vi "AddAutoMode.vi"(7 "error in (no error)":errorcluster, 9 "Autonomous Mode":string, 10 "Table Prefix":string="330AutonomousSelector") -> (0 "error out":errorcluster)   [LabVIEW 2012, in "AutonomousSelector.lvlib"]
doc: "Adds a single Autonomous Mode to the Autonomous Selector on the Dashboard. \n\n<B>Table Prefix</B> The Sub Table in Network Tables. The data will be stored in /SmartDashboard/<Table Prefix>\n<B>Autonomous Mode</B> The name of the Autonomous Mode to add"
uses:
  AutonomousSelector.lvlib
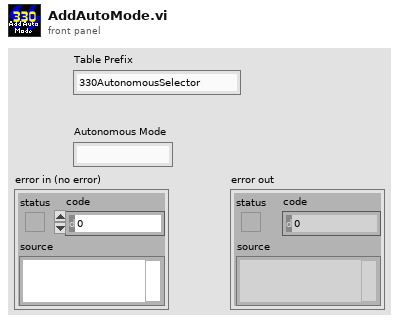
[diagram p1: front panel]
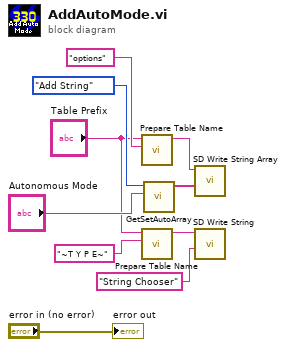
[diagram p0: block diagram]
diagram:
  n1 = call <vilib>:"Prepare Table Name.vi"("Name"="options", "Table Prefix"="Table Prefix") -> ("Prefixed Name"=w9:string)  [unwired: 9 in]
  n2 = call <vilib>:"Prepare Table Name.vi"("Name"="~T Y P E~", "Table Prefix"="Table Prefix") -> ("Prefixed Name"=w2:string)  [unwired: 9 in]
  n3 = call "GetSetAutoArray.vi"("String"="Autonomous Mode", "Mode"=enum16{"Get", "Add String", "Add String Array"}."Add String") -> ("Auto List"=w6:string[])  [unwired: 9 in]
  n4 = call <vilib>:"SD Write String Array.vi"("String Array"=w6, "Name"=w9) -> ()  [unwired: 8 in, 2 out]
  n5 = call <vilib>:"SD Write String.vi"("String"="String Chooser", "Name"=w2) -> ()  [unwired: 8 in, 2 out]
  "error out" <- "error in (no error)"
